vi "超标留样启动.vi"(8 "error in (no error)":errorcluster) -> (0 "error out":errorcluster)   [LabVIEW 2016, in "超标留样集成.lvlib" / "科盛超标留样.lvlib"]
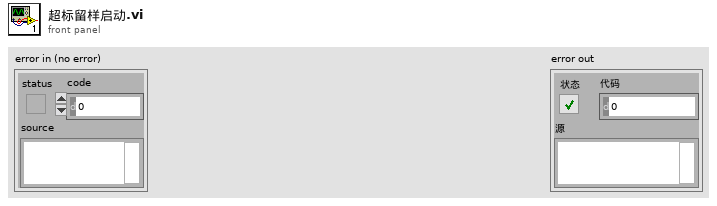
[diagram p1: front panel]
types:
  T1 = cluster{"STEP":enum16{"open", "read", "write", "close"}, "写入缓冲区":string}
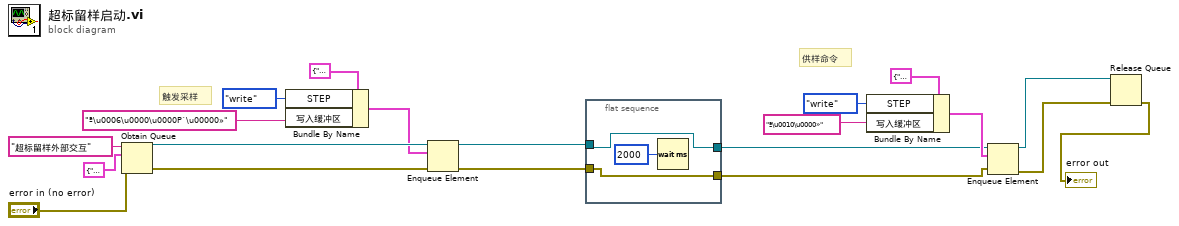
[diagram p0: block diagram]
diagram:
  # "供样命令"
  # "触发采样"
  n1 = Obtain Queue(name (unnamed)="超标留样外部交互" ("名称（未命名）"), element data type=T1 {"STEP"=enum."write", "写入缓冲区"="ª\u0006\u0000\u0000P`\u00000»"}, error in (no error)="error in (no error)") -> (queue out=w18:refnum<queue>, error out=w17:errorcluster)  [unwired: 2 in, 1 out]
  n2 = Bundle By Name(cluster=T1 {"STEP"=enum."open", "写入缓冲区"=""} ("元素"), "STEP"=enum16{"open", "read", "write", "close"}."write", "写入缓冲区"="ª\u0006\u0000\u0000P`\u00000»") -> (w14:T1)
  n3 = Enqueue Element(queue=w18, element=w14, error in (no error)=w17) -> (queue out=w7:refnum<queue>, error out=w5:errorcluster)  [unwired: 1 in, 1 out]
  n4 = flat-sequence {
    tunnel: w7 -> [w22]
    tunnel: [w22] -> w6
    tunnel: w5 -> [w21]
    tunnel: [w21] -> w4
    frame #0 {
      n5 = Wait (ms)(milliseconds to wait=u32 2000 ("等待时间（毫秒）")) -> ()  [unwired: 1 out]
    }
  }
  n6 = Bundle By Name(cluster=T1 {"STEP"=enum."open", "写入缓冲区"=""} ("元素"), "STEP"=enum16{"open", "read", "write", "close"}."write", "写入缓冲区"="ª\u0010\u0000»") -> (w9:T1)
  n7 = Enqueue Element(queue=w6, element=w9, error in (no error)=w4) -> (queue out=w1:refnum<queue>, error out=w3:errorcluster)  [unwired: 1 in, 1 out]
  n8 = Release Queue(queue=w1, error in (no error)=w3) -> (error out=→"error out":errorcluster)  [unwired: 1 in, 2 out]
